vi "MenuHandler.vi"(5 "tree control":refnum<vi>, 7 "main message queue":T1, 8 "error in":errorcluster, 9 "parameters":variant, 10 "menu string":string, 11 "NISE_CEF_serializable node in":refnum<class "NISE_CEF_serializable node.lvclass">) -> (0 "error out":errorcluster, 2 "Unhandled":bool, 3 "NISE_CEF_serializable node out":refnum<class "NISE_CEF_serializable node.lvclass">)   [LabVIEW 2013, in "NISE_CEF_serializable node.lvclass"]
uses:
  NISE_CEF_serializable node.lvclass
  <vilib>/NI/AMC/Message Queue.ctl
  <vilib>/NI/AMC/Message.ctl
  <vilib>/NI/Tools/Keyed Array/KeyedArray.ctl
  Node/NISE_CEF_Node.lvclass
  <vilib>/NI/Tools/Keyed Array/Tools_KeyedArray.lvlib
  <vilib>/NI/AMC/AMC.lvlib
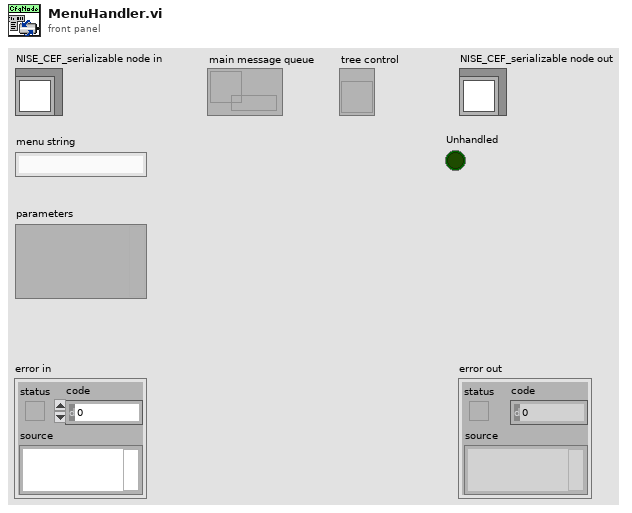
[diagram p1: front panel]
types:
  T1 = typedef "AMC.lvlib/Message Queue.ctl" = refnum<queue>
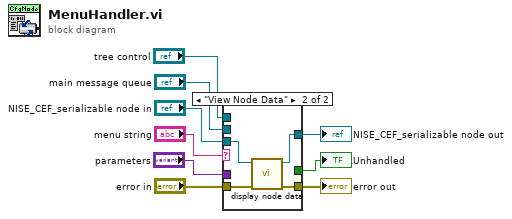
[diagram p0: block diagram]
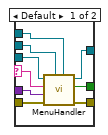
[diagram p2: hidden frame]
diagram:
  n1 = case shown="\"View Node Data\"" "menu string" {
    selector: "menu string" -> [w10 _]
    tunnel: [w16 _] -> w5
    tunnel: "NISE_CEF_serializable node in" -> [w14 w22]
    tunnel: [w13 w21] -> w8
    tunnel: [w17 w20] -> w4
    tunnel: "error in" -> [w18 w19]
    tunnel: "main message queue" -> [w15 _]
    tunnel: "parameters" -> [w12 _]
    tunnel: "tree control" -> [w11 _]
    frame Default {
      n2 = call-parent "MenuHandler.vi"("tree control"=w11, "main message queue"=w15, "error in"=w18, "parameters"=w12, "menu string"=w10, "NISE_CEF_Node in"=w14) -> ("error out"=w17:errorcluster, "Unhandled"=w16:bool, "NISE_CEF_Node out"=w13:refnum<class "NISE_CEF_serializable node.lvclass">)  [unwired: 3 in]
    }
    frame "View Node Data" {
      n3 = call-dynamic "display node data.vi"("error in"=w19, "NISE_CEF_serializable node in"=w22) -> ("error out"=w20:errorcluster, "NISE_CEF_serializable node out"=w21:refnum<class "NISE_CEF_serializable node.lvclass">)  [unwired: 8 in]
    }
  }
  "error out" <- w4
  "NISE_CEF_serializable node out" <- w8
  "Unhandled" <- w5
